vi "MyReadMagField1.vi"(8 "error in (no error)":errorcluster, 11 "VISA resource name in":refnum<visa-resource-name>="TCPIP0::192.168.0.107::33576::SOCKET") -> (0 "error out":errorcluster, 1 "B":dbl, 3 "VISA resource name out":refnum<visa-resource-name>)   [LabVIEW 2025]
uses:
  MyTriton.lvlib
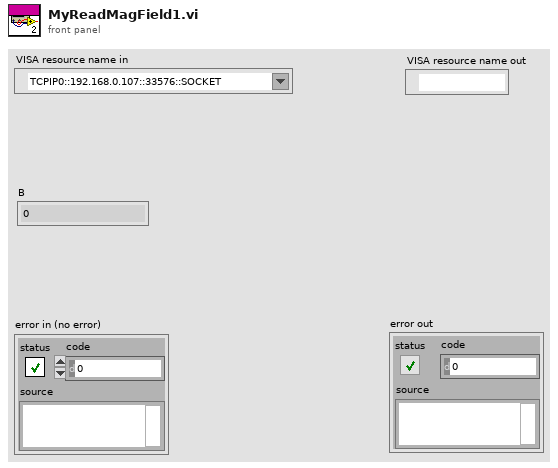
[diagram p1: front panel]
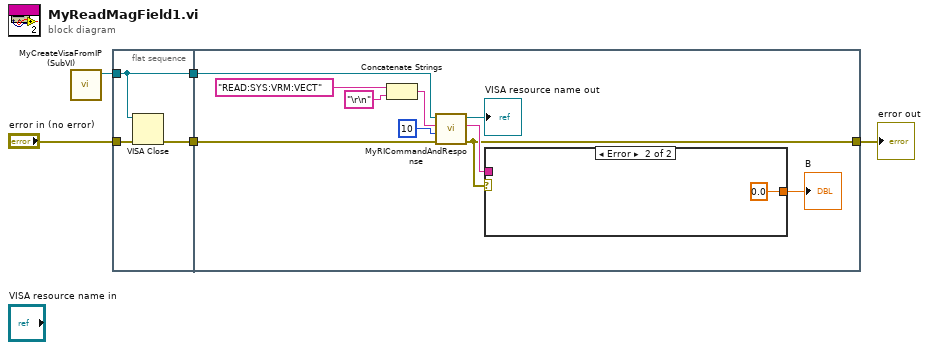
[diagram p0: block diagram]
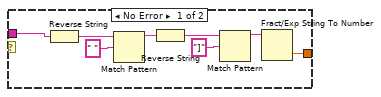
[diagram p2: hidden frame]
diagram:
  n1 = call "MyCreateVisaFromIP (SubVI).vi"() -> ("VISA Refnum out"=w5:refnum<visa-resource-name>)  [unwired: 11 in]
  n2 = flat-sequence {
    tunnel: w5 -> [w6]
    tunnel: "error in (no error)" -> [w8]
    tunnel: [w7] -> w3
    tunnel: [w6] -> w2
    tunnel: w3 -> [w11]
    tunnel: w2 -> [w10]
    tunnel: [w9] -> w1
    frame #0 {
      n3 = VISA Close(VISA resource name=w6, error in (no error)=w8) -> (error out=w7:errorcluster)
    }
    frame #1 {
      n4 = Concatenate Strings("READ:SYS:VRM:VECT" ("Command"), "\r\n" ("string")) -> (w16:string)
      n5 = call "MyRICommandAndResponse.vi"("error in (no error)"=w11, "Min byte count"=u32 10 ("byte count"), "Command"=w16, "VISA resource name in"=w10) -> ("error out"=w9:errorcluster, "Response"=w13:string, "VISA resource name out"=→"VISA resource name out":refnum<visa-resource-name>)  [unwired: 5 in]
      n6 = case shown="Error" w9 {
        tunnel: w13 -> [w23 _]
        tunnel: [w19 0.0] -> w12
        frame No Error {
          n7 = Reverse String(1:w23) -> (0:w26:string)
          n8 = Match Pattern(string=w26, regular expression=" ") -> (before substring=w24:string)  [unwired: 1 in, 3 out]
          n9 = Reverse String(1:w24) -> (0:w22:string)
          n10 = Match Pattern(string=w22, regular expression="]") -> (before substring=w20:string)  [unwired: 1 in, 3 out]
          n11 = Fract/Exp String To Number(string=w20) -> (number=w19:dbl)  [unwired: 3 in, 1 out]
        }
        frame Error {
        }
      }
      "B" <- w12
    }
  }
  "error out" <- w1
